vi "Recursive XML Parse.vi"(7 "Parent ID":string, 8 "error in (no error)":errorcluster, 10 "DOM document in":refnum<k20>, 11 "Tree":refnum<data-value>) -> (0 "error out":errorcluster, 3 "Tree Manager":refnum<data-value>)   [LabVIEW 2016]
uses:
  <vilib>/ni/Tree/Tree Manager/Tree.lvclass
  <resource>/objmgr/DOMUserDefRef.rc
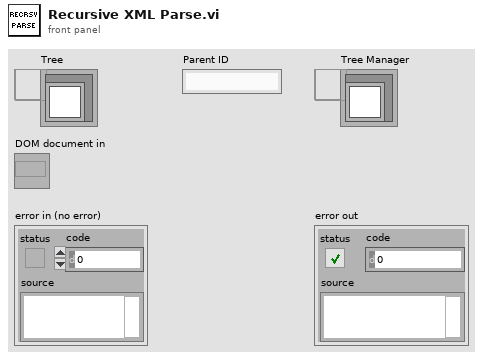
[diagram p1: front panel]
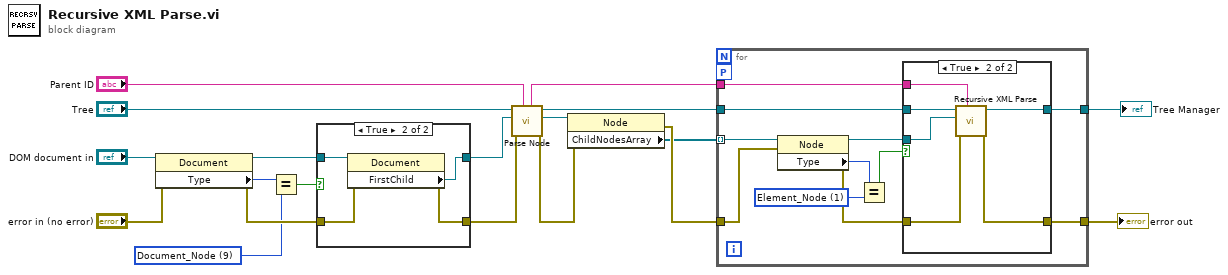
[diagram p0: block diagram]
diagram:
  w3 = 9 items=["Element_Node"=1, "Attribute_Node"=2, "Text_Node"=3, "CDATASection_Node"=4, "EntityReference_Node"=5, "Entity_Node"=6, "ProcessingInstruction_Node"=7, "Comment_Node"=8, "Document_Node"=9, "DocumentType_Node"=10, "DocumentFragment_Node"=11, "Notation_Node"=12] ("Node Type")
  n1 = property class="Document"(reference="DOM document in", error in="error in (no error)") -> (reference out=w5:refnum<k20>, error out=w15:errorcluster, "Type"=w4:i32)
  n2 = Equal?(x=w4, y=w3) -> (x = y?=w1:bool)
  n3 = case shown="True" w1 {
    tunnel: w5 -> [w20 w23]
    tunnel: [w20 w22] -> w2
    tunnel: w15 -> [w21 w25]
    tunnel: [w21 w24] -> w14
    frame False {
    }
    frame True {
      n4 = property class="Document"(reference=w23, error in=w25) -> (error out=w24:errorcluster, "FirstChild"=w22:refnum<k20>)  [unwired: 1 out]
    }
  }
  n5 = call "Parse Node.vi"("Parent ID"="Parent ID", "error in (no error)"=w14, "Node in"=w2, "Tree in"="Tree") -> ("error out"=w19:errorcluster, "Node out"=w10:refnum<k20>, "Tree out"=w8:refnum<data-value>, "Unique ID"=w7:string)  [unwired: 4 in]
  n6 = property class="Node"(reference=w10, error in=w19) -> (error out=w18:errorcluster, "ChildNodesArray"=w9:refnum<k20>[])  [unwired: 1 out]
  n7 = for {
    tunnel: w9 -> [w31] mode=indexing
    tunnel: w7 -> [w32]
    workers-P: _ -> [_]
    tunnel: w18 -> [w35]
    tunnel: [w36] -> w17
    tunnel: w8 -> [w33]
    tunnel: [w30] -> w6
    w27 = 1 items=["Element_Node"=1, "Attribute_Node"=2, "Text_Node"=3, "CDATASection_Node"=4, "EntityReference_Node"=5, "Entity_Node"=6, "ProcessingInstruction_Node"=7, "Comment_Node"=8, "Document_Node"=9, "DocumentType_Node"=10, "DocumentFragment_Node"=11, "Notation_Node"=12] ("Node Type")
    n8 = property class="Node"(reference=w31, error in=w35) -> (reference out=w29:refnum<k20>, error out=w34:errorcluster, "Type"=w28:i32)
    n9 = Equal?(x=w28, y=w27) -> (x = y?=w26:bool)
    n10 = case shown="True" w26 {
      tunnel: w33 -> [w37 w42]
      tunnel: w32 -> [_ w41]
      tunnel: [w37 w40] -> w30
      tunnel: [w38 w44] -> w36
      tunnel: w29 -> [_ w39]
      tunnel: w34 -> [w38 w43]
      frame False {
      }
      frame True {
        n11 = call "Recursive XML Parse.vi"("Parent ID"=w41, "error in (no error)"=w43, "DOM document in"=w39, "Tree"=w42) -> ("error out"=w44:errorcluster, "Tree Manager"=w40:refnum<data-value>)  [unwired: 6 in]
      }
    }
  }
  "error out" <- w17
  "Tree Manager" <- w6
